vi "Task1.vi"() -> ()   [LabVIEW 2021]
uses:
  <vilib>/myRIO/Instrument Drivers/Onboard IO/DIO/typedefs/DIO Reference.ctl
  <vilib>/myRIO/Common/Instrument Driver Framework/Utilities/typedefs/myRIO Generic Hardware Reference.ctl
  <vilib>/myRIO/Common/Instrument Driver Framework/Utilities/typedefs/Hardware Version Enum.ctl
  <vilib>/myRIO/Common/Instrument Driver Framework/Utilities/typedefs/myRIO v1.0 Reference.ctl
  <vilib>/myRIO/Common/Instrument Driver Framework/Utilities/typedefs/Generic FPGA Reference.ctl
  <vilib>/myRIO/Common/Instrument Driver Framework/myRIO v1.0/DIO/typedefs/DIO Channels List.ctl
  <vilib>/myRIO/Common/Instrument Driver Framework/myRIO v1.0/DIO/typedefs/DIO Channels Enum.ctl
  <vilib>/userDefined/High Color/nirio_resource_hc.ctl
  <vilib>/myRIO/Common/Instrument Driver Framework/myRIO v1.0/DIO/vis/myRIO v1.1 Open DIO.vi
  <vilib>/myRIO/Common/Instrument Driver Framework/Utilities/vis/Validate Channels.vi
  <vilib>/myRIO/Common/Instrument Driver Framework/myRIO v1.0/DIO/vis/myRIO v1.0 Reserve DIO.vi
  <vilib>/myRIO/Common/Instrument Driver Framework/myRIO v1.0/DIO/vis/myRIO v1.0 Close DIO.vi
  <vilib>/myRIO/Common/Instrument Driver Framework/myRIO v1.0/Resource Manager/vis/myRIO v1.0 Reserve Channel List.vi
  <vilib>/myRIO/Common/Instrument Driver Framework/myRIO v1.0/DIO/vis/myRIO v1.0 Build MUX Configuration DIO.vi
  <vilib>/myRIO/Common/Instrument Driver Framework/myRIO v1.0/DIO/vis/myRIO v1.0 Unreserve DIO.vi
  <vilib>/myRIO/Common/Instrument Driver Framework/myRIO v1.0/Resource Manager/vis/myRIO v1.0 Reserve Channel.vi
  <vilib>/myRIO/Common/Instrument Driver Framework/myRIO v1.0/Resource Manager/vis/myRIO v1.0 Unreserve Channel.vi
  <vilib>/myRIO/Common/Instrument Driver Framework/myRIO v1.0/Resource Manager/vis/myRIO v1.0 Create Configuration List.vi
  <vilib>/myRIO/Common/Instrument Driver Framework/myRIO v1.0/Resource Manager/vis/myRIO v1.0 Unreserve Channel List.vi
  <vilib>/myRIO/Common/Instrument Driver Framework/myRIO v1.0/Resource Manager/vis/myRIO v1.0 Build Mutex Name.vi
  <vilib>/Utility/VariantDataType/GetNumericInfo.vi
  <vilib>/Utility/error.llb/Error Cluster From Error Code.vi
  <vilib>/myRIO/Common/Instrument Driver Framework/myRIO v1.0/myRIO v1.1 Open.vi
  <vilib>/myRIO/Common/Instrument Driver Framework/Utilities/vis/IO Manager.vi
  <vilib>/myRIO/Common/Instrument Driver Framework/Utilities/vis/Configuration Manager.vi
  <vilib>/myRIO/Common/Instrument Driver Framework/myRIO v1.0/Resource Manager/vis/myRIO v1.0 Configure IO.vi
  <vilib>/myRIO/Common/Instrument Driver Framework/myRIO v1.0/myRIO v1.0 Close.vi
  <vilib>/myRIO/Common/Instrument Driver Framework/myRIO v1.0/DIO/vis/myRIO v1.0 Write DIO.vi
  <vilib>/myRIO/Common/Instrument Driver Framework/myRIO v1.0/DIO/vis/myRIO v1.0 Shutdown DIO.vi
  <vilib>/myRIO/Instrument Drivers/Onboard IO/DIO/vis/myRIO DIO Open.xnode
  <vilib>/myRIO/Instrument Drivers/Onboard IO/DIO/DIO.lvlib
panel:
  in  "stop":bool
  in  "RPM":dbl(slide) scale=10.0..1000.0
  out "Visualize":bool[](array[boolean])
  in  "Full Step":bool
  in  "Direction":enum32{"CW", "CCW"}(radio)
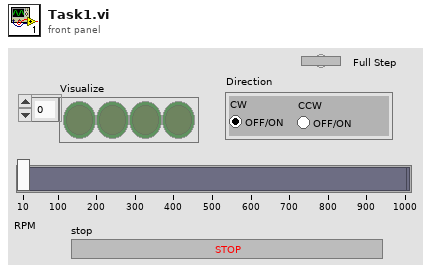
[diagram p1: front panel]
types:
  T1 = typedef "DIO.lvlib/DIO Reference.ctl" = cluster{"myRIO Reference":T2, "DIO Channels List":T6}
  T2 = typedef "myRIO Generic Hardware Reference.ctl" = cluster{"myRIO Model":T3, "myRIO Hardware Reference":T4}
  T3 = typedef "Hardware Version Enum.ctl" = enum16{"Unknown", "myRIO-1900", "myRIO-1950", "roboRIO", "NI ELVIS RIO CM", "ELVIS III"}
  T4 = typedef "myRIO v1.0 Reference.ctl" = cluster{"Generic FPGA Reference":T5, "Allow multiple opens":bool}
  T5 = typedef "Generic FPGA Reference.ctl" = refnum<k20>
  T6 = typedef "DIO Channels List.ctl" = T7[]
  T7 = typedef "DIO Channels Enum.ctl" = enum16{"Not Connected", "C/DIO0", "C/DIO1", "C/DIO2", "C/DIO3", "C/DIO4", "C/DIO5", "C/DIO6", "C/DIO7", "A/DIO0", "A/DIO1", "A/DIO2", "A/DIO3", "A/DIO4", "A/DIO5", "A/DIO6", "A/DIO7", "A/DIO8", "A/DIO9", "A/DIO10", "A/DIO11", "A/DIO12", "A/DIO13", "A/DIO14", "A/DIO15", "A/DIO16", "A/DIO17", "A/DIO18", "A/DIO19", "B/DIO0", "B/DIO1", "B/DIO2", "B/DIO3", "B/DIO4", "B/DIO5", "B/DIO6", "B/DIO7", "B/DIO8", "B/DIO9", "B/DIO10", "B/DIO11", "B/DIO12", "B/DIO13", "B/DIO14", "B/DIO15", "B/DIO16", "B/DIO17", "B/DIO18", "B/DIO19", "LED0", "LED1", "LED2", "LED3", "Button0", "DIO/DIO0", "DIO/DIO1", "DIO/DIO2", "DIO/DIO3", "DIO/DIO4", "DIO/DIO5", "DIO/DIO6", "DIO/DIO7", "DIO/DIO8", "DIO/DIO9", "SPI/CS0", "SPI/CS1", "SPI/CS2", "SPI/CS3", "LED RADIO (Green)", "LED RADIO (Red)", "LED COMM (Green)", "LED COMM (Red)", "LED MODE (Green)", "LED MODE (Red)"}
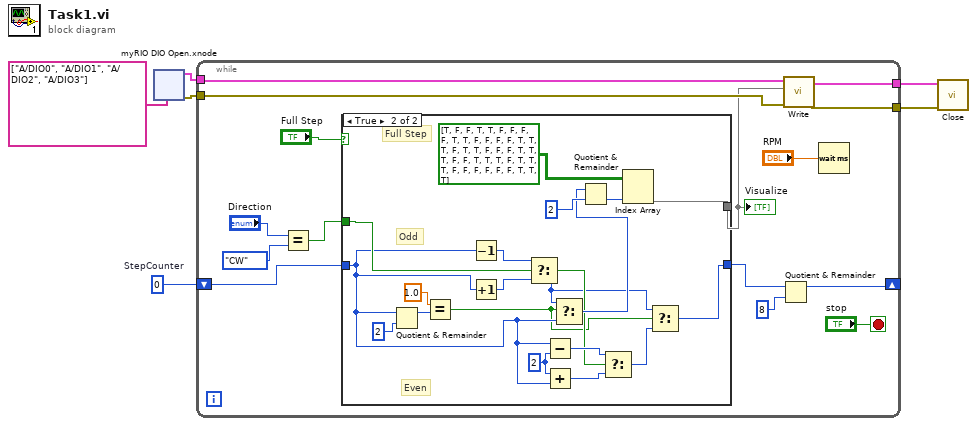
[diagram p0: block diagram]
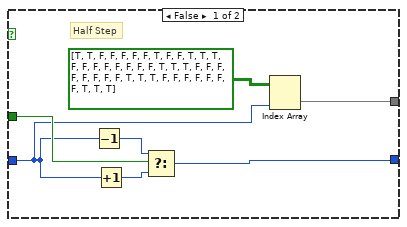
[diagram p2: hidden frame]
diagram:
  w5 = 0  # StepCounter
  n1 = xnode "myRIO DIO Open.xnode"("Channel Names"=tag[] ["A/DIO0", "A/DIO1", "A/DIO2", "A/DIO3"]) -> ("error out"=w4:errorcluster, "DIO Ref Out"=w3:T1)  [unwired: 2 in]
  n2 = while {
    shift-right: [w15] -> _
    shift-left: w5 -> [w18]
    tunnel: w4 -> [w10]
    tunnel: w3 -> [w11]
    tunnel: [w8] -> w2
    tunnel: [w7] -> w1
    stop <- "stop" stop-if-true
    n3 = Equal?(x="Direction", y=enum32{"CW", "CCW"}."CW") -> (x = y?=w12:bool)
    n4 = case shown="True" "Full Step" {
      tunnel: w18 -> [w22 w33]
      tunnel: [w24 w29] -> w17
      tunnel: w12 -> [w28 w35]
      tunnel: [w27 w37] -> w9
      frame False {
        # "Half Step"
        n5 = Decrement(x=w22) -> (x-1=w26:i32)
        n6 = Increment(x=w22) -> (x+1=w25:i32)
        n7 = Select(t=w26, s=w28, f=w25) -> (s? t:f=w24:i32)
        n8 = Index Array(array=bool[][] [[TRUE, TRUE, FALSE, FALSE, FALSE, FALSE, FALSE, TRUE, FALSE], [FALSE, TRUE, TRUE, TRUE, FALSE, FALSE, FALSE, FALSE, FALSE], [FALSE, FALSE, FALSE, TRUE, TRUE, TRUE, FALSE, FALSE, FALSE], [FALSE, FALSE, FALSE, FALSE, FALSE, TRUE, TRUE, TRUE, FALSE], [FALSE, FALSE, FALSE, FALSE, FALSE, FALSE, TRUE, TRUE, TRUE]], index (col)=w22) -> (element=w27:bool[])  [unwired: 1 in]
      }
      frame True {
        w47 = 2 ("y")
        # "Odd"
        # "Even"
        # "Full Step"
        n9 = Quotient & Remainder(x=w33, y=2) -> (x-y*floor(x/y)=w43:i32)  [unwired: 1 out]
        n10 = Equal?(x=1.0, y=w43) -> (x = y?=w32:bool)
        n11 = Decrement(x=w33) -> (x-1=w42:i32)
        n12 = Increment(x=w33) -> (x+1=w41:i32)
        n13 = Select(t=w42, s=w35, f=w41) -> (s? t:f=w31:i32)
        n14 = Subtract(x=w33, y=w47) -> (x-y=w46:i32)
        n15 = Add(x=w47, y=w33) -> (x+y=w40:i32)
        n16 = Select(t=w31, s=w32, f=w33) -> (s? t:f=w36:i32)
        n17 = Quotient & Remainder(x=w36, y=2) -> (floor(x/y)=w34:i32)  [unwired: 1 out]
        n18 = Select(t=w46, s=w35, f=w40) -> (s? t:f=w30:i32)
        n19 = Index Array(array=bool[][] [[TRUE, FALSE, FALSE, TRUE, TRUE, FALSE, FALSE, FALSE, FALSE], [TRUE, TRUE, FALSE, FALSE, FALSE, FALSE, TRUE, TRUE, TRUE], [FALSE, TRUE, TRUE, FALSE, FALSE, FALSE, TRUE, TRUE, TRUE], [FALSE, FALSE, TRUE, TRUE, TRUE, FALSE, TRUE, TRUE, TRUE], [FALSE, FALSE, FALSE, FALSE, FALSE, FALSE, TRUE, TRUE, TRUE]], index (col)=w34) -> (element=w37:bool[])  [unwired: 1 in]
        n20 = Select(t=w31, s=w32, f=w30) -> (s? t:f=w29:i32)
      }
    }
    "Visualize" <- w9
    n21 = Quotient & Remainder(x=w17, y=8) -> (x-y*floor(x/y)=w15:i32)  [unwired: 1 out]
    n22 = call <vilib>:"Write.vi"("error in (no error)"=w10, "Values"=w9, "DIO Ref In"=w11) -> ("error out"=w7:errorcluster, "DIO Ref Out"=w8:T1)  [unwired: 6 in]
    n23 = Wait (ms)(milliseconds to wait="RPM") -> ()  [unwired: 1 out]
  }
  n24 = call <vilib>:"Close.vi"("error in (no error)"=w1, "DIO Ref In"=w2) -> ()  [unwired: 9 in, 1 out]
